vi "Calculate and Draw Picture.vi"(9 "Draw Circle?":bool, 10 "Time":dbl, 11 "Inputs":T1[](array[typedef])) -> (2 "Points":cluster{dbl[], dbl[]}[](array[cluster]), 3 "Endpoint":cluster{"x":dbl, "y":dbl})   [LabVIEW 2020]
uses:
  Component.ctl
  <vilib>/gmath/NI_Gmath.lvlib
panel:
  out "XY Graph":cluster{dbl[], dbl[]}[](graph)
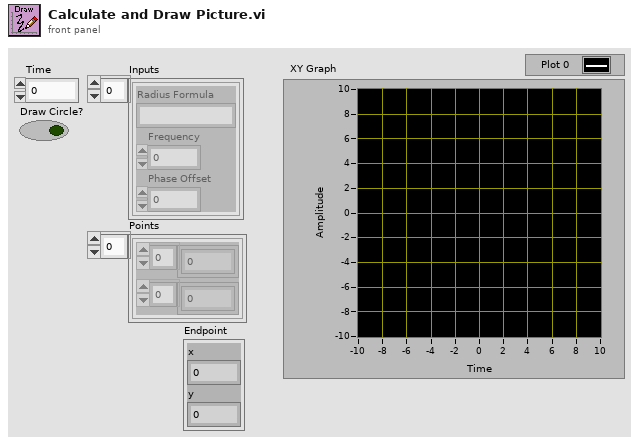
[diagram p1: front panel]
types:
  T1 = typedef "Component.ctl" = cluster{"Radius Formula":string, "Frequency":dbl, "Phase Offset":dbl}
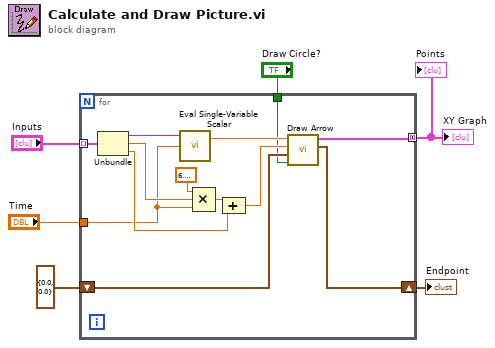
[diagram p0: block diagram]
diagram:
  n1 = for {
    tunnel: "Inputs" -> [w19] mode=indexing
    tunnel: "Time" -> [w8]
    shift-right: [w14] -> w2
    shift-left: cluster{"x":dbl, "y":dbl} {"x"=0.0, "y"=0.0} ("Offset") -> [w13]
    tunnel: [w12] -> w3 mode=concatenating
    tunnel: "Draw Circle?" -> [w11]
    n2 = Unbundle(w19) -> ("Radius Formula"=w18:string, "Frequency"=w9:dbl, "Phase Offset"=w17:dbl)
    n3 = call <vilib>:"Eval Single-Variable Scalar.vi"("x value"=w8, "formula"=w18) -> ("y value"=w15:dbl)  [unwired: 1 in, 1 out]
    n4 = Compound Arithmetic op=MULTIPLY(6.283185307179586, w9, w8) -> (w10:dbl)
    n5 = Compound Arithmetic op=ADD(w10, w17) -> (w16:dbl)
    n6 = call "Draw Arrow.vi"("Draw Circle?"=w11, "Offset"=w13, "Theta"=w16, "Radius"=w15) -> ("Endpoint"=w14:cluster{dbl, dbl}, "Points"=w12:cluster{dbl[], dbl[]}[])  [unwired: 6 in]
  }
  "XY Graph" <- w3
  "Endpoint" <- w2
  "Points" <- w3
